vi "Process.vi"(8 "error in":errorcluster, 11 "Instrument.OxfordVRM UI.lvclass":refnum<class "Instrument.OxfordVRM UI.lvclass">) -> (0 "error out":errorcluster, 3 "Instrument.OxfordVRM UI.lvclass":refnum<class "Instrument.OxfordVRM UI.lvclass">)   [LabVIEW 2016, in "Instrument.OxfordVRM UI.lvclass"]
doc: "---------------------------------------------------------------\nJKI State Machine Objects™\nhttp://jki.net/state-machine-objects/\nCopyright (C) 2005-2015, JKI <info@jki.net>\nALL RIGHTS RESERVEDJKI State Machine Objects (SMO) 1.0.0.5\nJKI - JKI\nCopyright (c) 2016, JKI"
uses:
  Instrument.OxfordVRM UI.lvclass
  <vilib>/JKI/JKI SMO/SMO/SMO.lvclass
  <vilib>/JKI/JKI SMO/SMO/Typedefs/Parent Call--Enum.ctl
  <vilib>/JKI/JKI SMO/SMO.UI/SMO.UI.lvclass
  <userlib>/LevyLab/Levylab Instruments/SMOs/Instrument/Instrument.lvclass
  Instrument.OxfordVRM/Typedefs/getAll.ctl
  Instrument.OxfordVRM/Instrument.OxfordVRM.lvclass
  <userlib>/LevyLab/Levylab Instruments/SMOs/Instrument UI/Instrument UI.lvclass
  C:/Program Files (x86)/National Instruments/LabVIEW 2016/user.lib/LevyLab/Levylab Instruments/SMOs/Instrument UI/Instrument UI.lvclass
  C:/Program Files (x86)/National Instruments/LabVIEW 2016/vi.lib/JKI/JKI SMO/SMO.UI/SMO.UI.lvclass
  C:/Program Files (x86)/National Instruments/LabVIEW 2016/vi.lib/JKI/JKI SMO/SMO/SMO.lvclass
  C:/Program Files (x86)/National Instruments/LabVIEW 2016/user.lib/LevyLab/Levylab Instruments/Instrument Types/Cryostat/Instrument.Cryostat.lvclass
  C:/Program Files (x86)/National Instruments/LabVIEW 2016/user.lib/LevyLab/Levylab Instruments/SMOs/Instrument/Instrument.lvclass
panel:
  out "Target Rate (T)":dbl[](array[numeric])
  out "Setpoint (T) (sph)":dbl[](array[numeric])
  in  "Setpoint (T)":dbl[](array[numeric])
  out "Field (T) (sph)":dbl[](array[numeric])
  out "Target Field (T) (sph)":dbl[](array[numeric])
  out "Target Field (T)":dbl[](array[numeric])
  out "Field (T)":dbl[](array[numeric])
  out "XY Graph":cluster{dbl[], dbl[]}[](graph)
  out "XZ Graph":cluster{dbl[], dbl[]}[](graph)
  out "Voltage Meter 6":dbl(knob) scale=-10.0..10.0
  out "Voltage Meter 5":dbl(knob) scale=-10.0..10.0
  out "Voltage Meter 4":dbl(knob) scale=-10.0..10.0
  out "Voltage Meter 3":dbl(knob) scale=-10.0..10.0
  out "Voltage Meter 2":dbl(knob) scale=-10.0..10.0
  out "Current Meter 6":dbl(knob) scale=-120.0..120.0
  out "Current Meter 5":dbl(knob) scale=-120.0..120.0
  out "Current Meter 4":dbl(knob) scale=-120.0..120.0
  out "Current Meter 3":dbl(knob) scale=-120.0..120.0
  out "Current Meter 2":dbl(knob) scale=-120.0..120.0
  out "Voltage Meter 1":dbl(knob) scale=-10.0..10.0
  out "Current Meter 1":dbl(knob) scale=-120.0..120.0
  out "System Time (HH:MM:SS)":dbl=165.3592643737793 format="%<%I:%M:%S %p>T"
  out "ETA":dbl=3660699600.0 format="%<%I:%M:%S %p %m/%d/%Y>T"
  out "version":string="v20/10/28"
  in  "Window Maximize":bool
  in  "Window Minimize":bool
  out "Magnet Status 3":string="Status: Clamped"
  in  "Hold":bool
  in  "To Set":bool
  in  "Export":bool
  in  "Target Field (T)":dbl caption="Field" format="%.2f"
  in  "Target Rate (T/min)":dbl=0.1 caption="Rate" min=0.0 max=1.0 format="%.2f"
  in  "To Zero":bool
  in  "Clamp":bool
  out "Magnet Status 2":string="Status: Clamped"
  in  "Power":bool
  # "Status"
  # "Actions"
  # "Targets"
  # "IPS"
  # "PSU 1 Current (A)"
  # "PSU 1 Voltage (V)"
  # "PSU 2 Current (A)"
  # "PSU 2 Voltage (V)"
  # "PSU 3 Current (A)"
  # "PSU 3 Voltage (V)"
  # "PSU 4 Current (A)"
  # "PSU 4 Voltage (V)"
  # "PSU 5 Current (A)"
  # "PSU 5 Voltage (V)"
  # "PSU 6 Current (A)"
  # "PSU 6 Voltage (V)"
  # "SMO UI Template"
  # "X \t\t\nCurrent (A)\tField (T)\t    Rate (T/min)\n0  - 30 \t   0    - 0.6 \t  0.06\n30 - 42\t    0.6  - 0.85\t  0.048\n42 - 60\t    0.85 - 1.2\t   0.042\n60 - 80\t    1.2  - 1.6\t   0.036\n80 - 99\t    1.6  - 2.0\t   0.024"
  # "Y \t\t\nCurrent (A)\tField (T)\t    Rate (T/min)\n0  - 30\t    0    - 0.6\t   0.048\n30 - 35\t    0.6  - 0.69\t  0.035\n35 - 45\t    0.69 - 0.89\t  0.03\n45 - 60\t    0.89 - 1.2\t   0.024\n60 - 80\t    1.2  - 1.58\t  0.018\n80 - 101\t   1.58 - 2\t     0.01"
  # "Z \t\t\nCurrent (A)\tField (T)\t    Rate (T/min)\n0  - 30\t    0    - 2.6    0.26\n30 - 60\t    2.6  - 5.3\t   0.21\n60 - 80\t    5.3  - 7.1\t   0.16\n80 - 90\t    7.1  - 8\t     0.13\n90 - 101\t   8    - 9\t     0.1\n\n2 OR MORE AXES\n0.005 T/min"
  # "For instructions on how to use the JKI State Machine Objects, examples and video tutorials, visit:\nhttp://jki.net/state-machine-objects/\n\nJKI State Machine Objects™\nhttp://jki.net/state-machine-objects/\nCopyright (C) 2005-2015, JKI <info@jki.net>\nALL RIGHTS RESERVED"
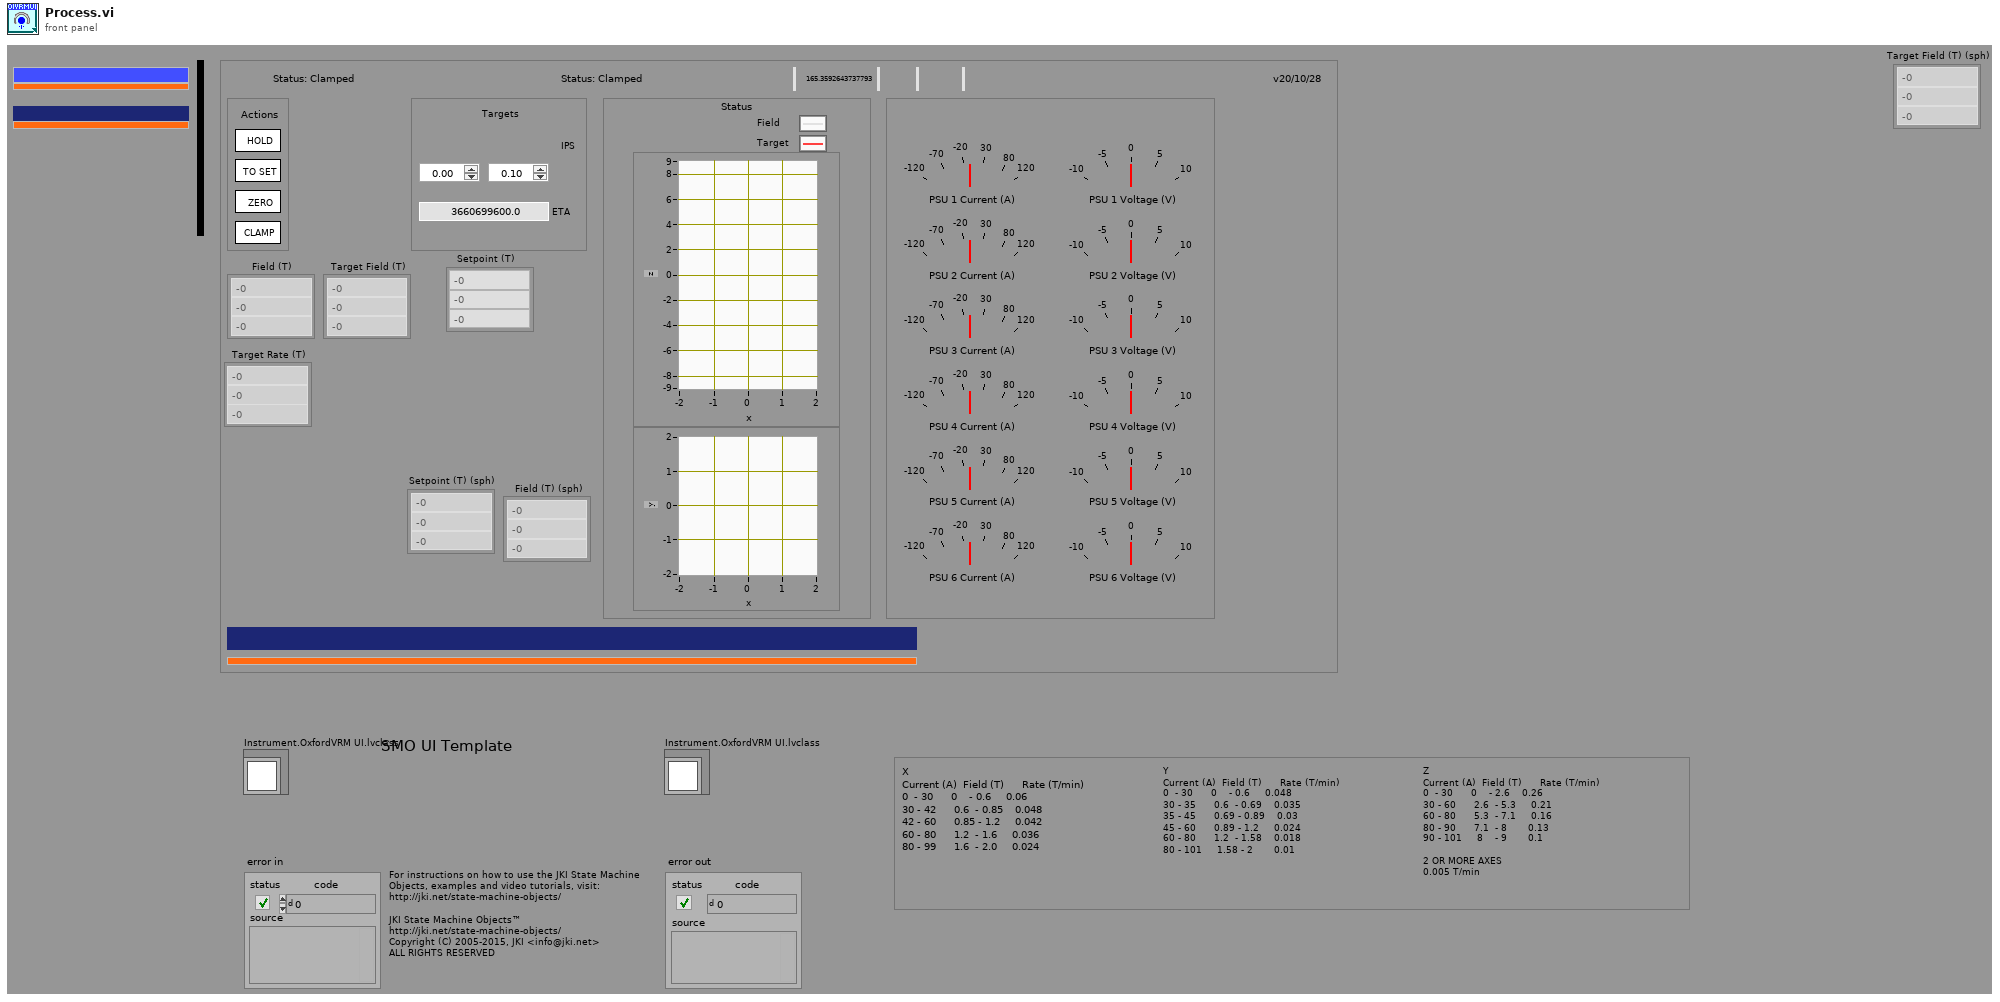
[diagram p1: front panel]
types:
  T1 = typedef "SMO.lvclass/Parent Call--Enum.ctl" = enum16{"Allows parent to run", "Does not request parent to run"}
  T2 = enum32{"invalid app kind", "Development System", "Run Time System", "Student Edition", "Embedded LabVIEW", "Evaluation", "Custom"}
  T3 = typedef "Instrument.OxfordVRM.lvclass/getAll.ctl" = cluster{"Field":dbl[], "Target Field":dbl[], "Target Field Rate":dbl[], "PSU Current":dbl[], "PSU Voltage":dbl[], "Status":string[]}
  T4 = enum32{"Invalid", "Standard", "Closed", "Hidden", "Minimized", "Maximized"}
  T5 = typedef "RemoteControl.lvclass/Message--Cluster.ctl" = cluster{"Command":string, "Data":variant, "Message ID":i32}
  T6 = cluster{"Core":cluster{"Current VI Reference":refnum<vi>, "Close Panel on Exit?":bool, "error":errorcluster}, "Instrument UI out":refnum<class "Instrument.OxfordVRM UI.lvclass">, "Instrument":refnum<class "Instrument.OxfordVRM.lvclass">, "getAll":variant, "Response":string, "config":variant, "switch time":timestamp, "LPF time":timestamp}
  T7 = typedef "Instrument.OxfordVRM.lvclass/PublicEvents--Instrument.Oxford1820.ProcessStatus.ctl" = string
  T8 = cluster{"Current VI Reference":refnum<vi>, "Close Panel on Exit?":bool, "error":errorcluster}
  T9 = typedef "LVRectTypeDef.ctl" = cluster{"Left":i16, "Top":i16, "Right":i16, "Bottom":i16}
  T10 = typedef "SMO.lvclass/Protected Events.ctl" = cluster{"StopProcesses":refnum<user-event>, "AbortProcesses":refnum<user-event>, "Config Changed":refnum<user-event>, "Dependency":refnum<user-event>}
  T11 = typedef "Instrument.lvclass/PublicEvents--Cluster.ctl" = cluster{"MessageFromProcess":refnum<user-event>}
  T12 = typedef "Instrument.OxfordVRM.lvclass/PublicEvents--Cluster.ctl" = cluster{"ProcessStatus":refnum<user-event>}
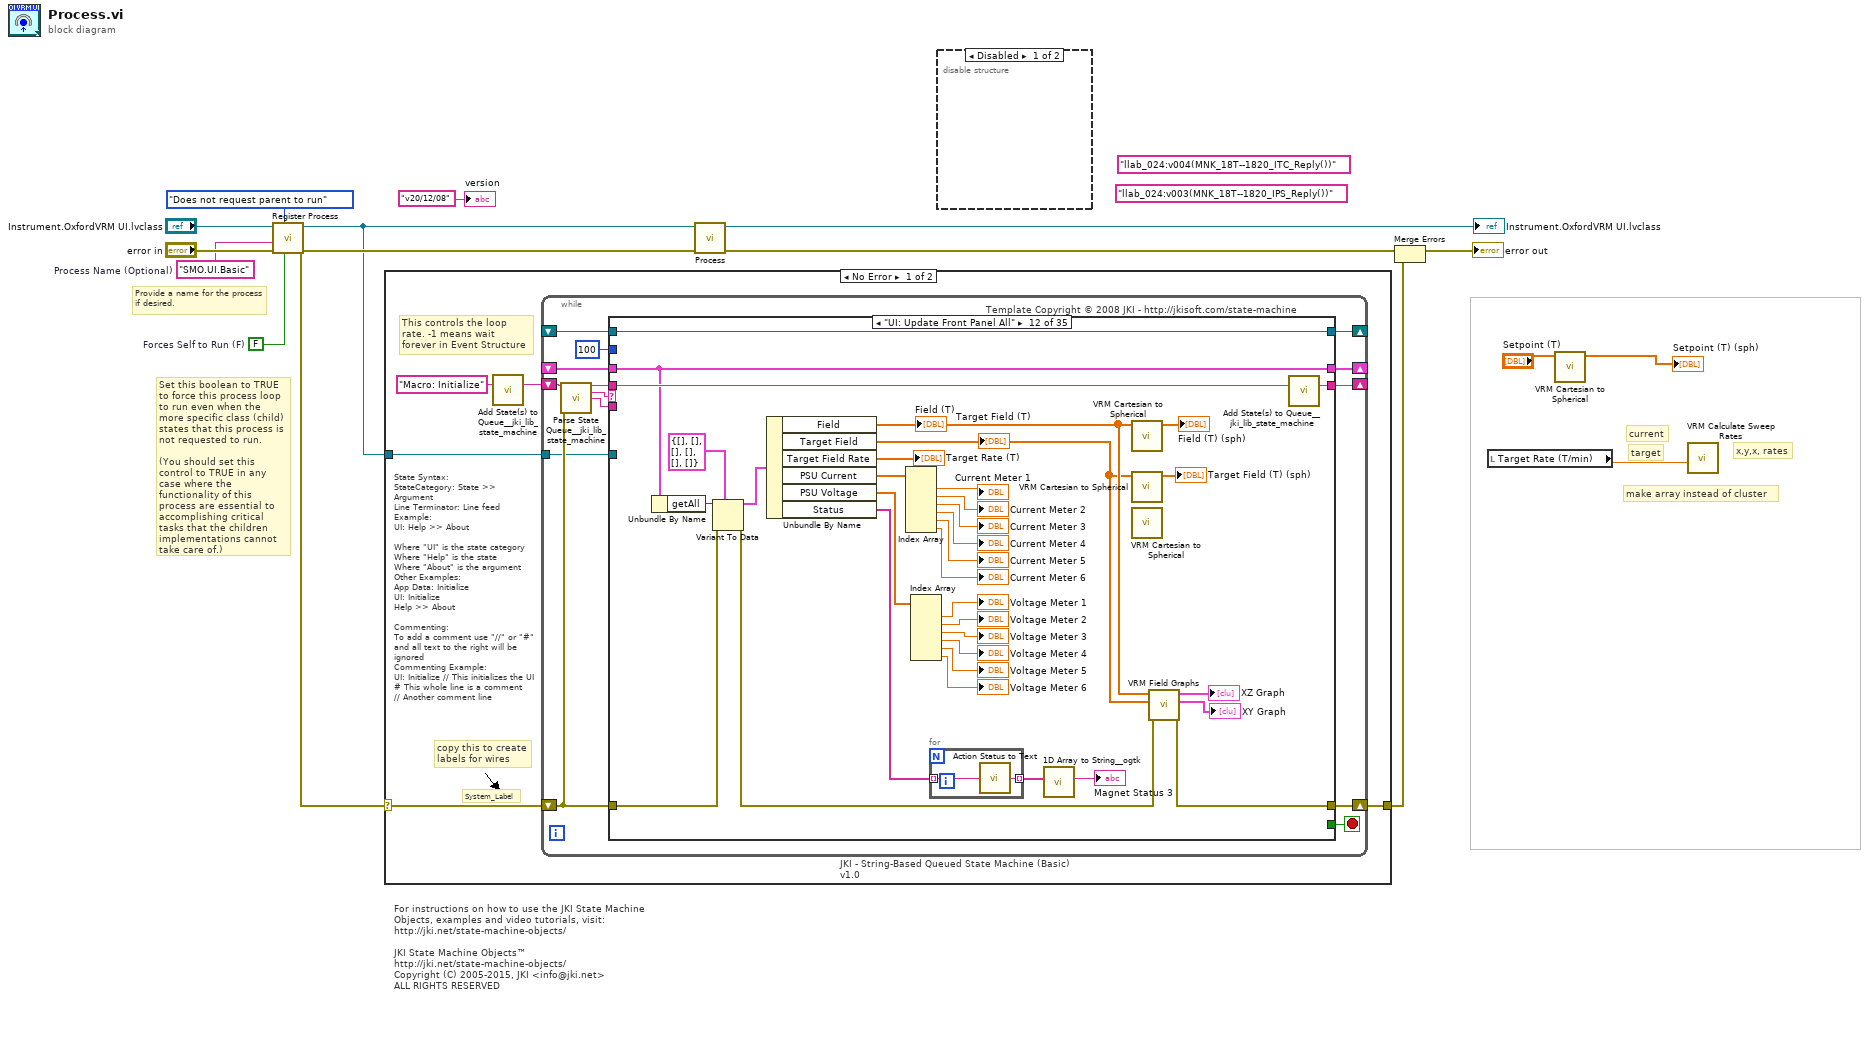
[diagram p0: block diagram]
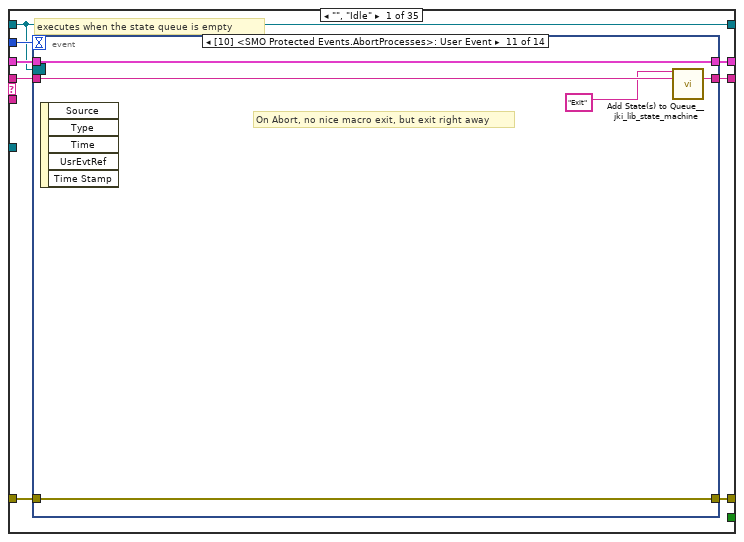
[diagram p3: hidden frame]
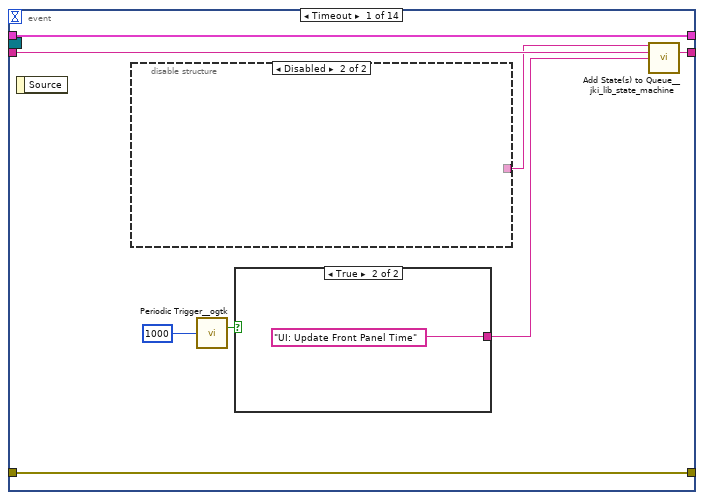
[diagram p4: hidden frame]
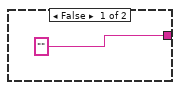
[diagram p5: hidden frame]
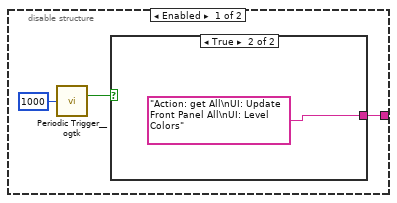
[diagram p6: hidden frame]
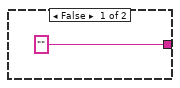
[diagram p7: hidden frame]
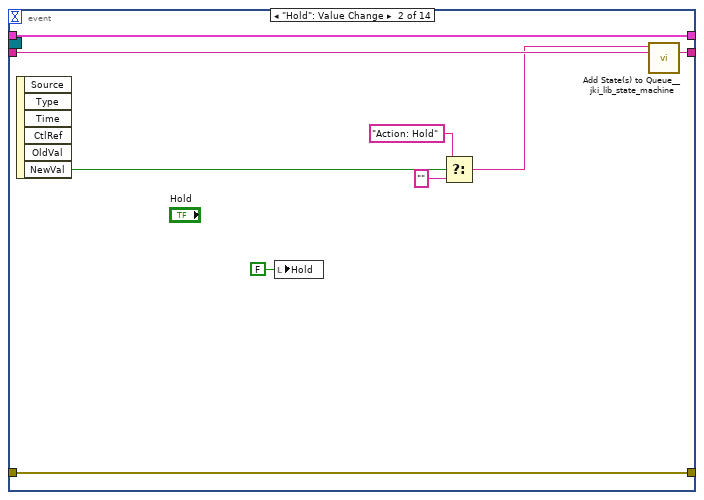
[diagram p8: hidden frame]
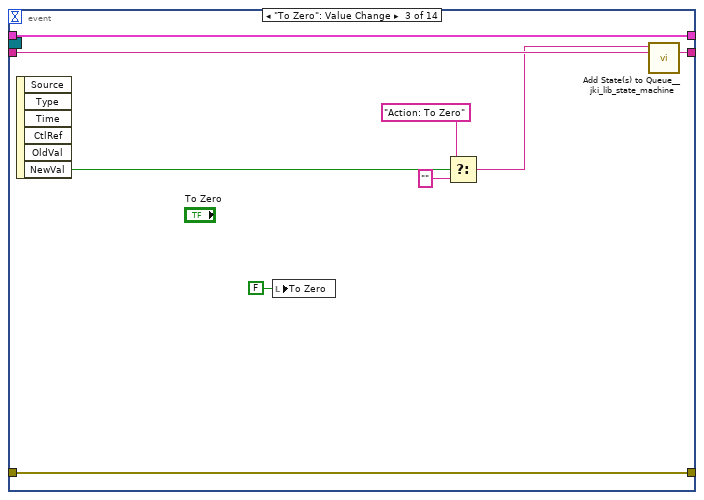
[diagram p9: hidden frame]
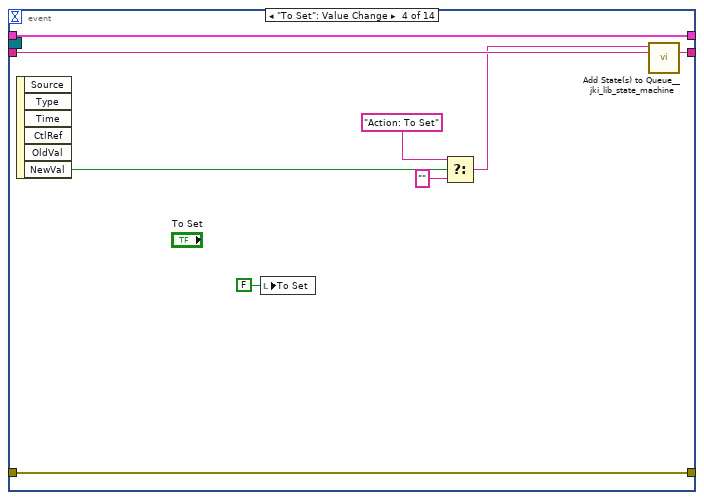
[diagram p10: hidden frame]
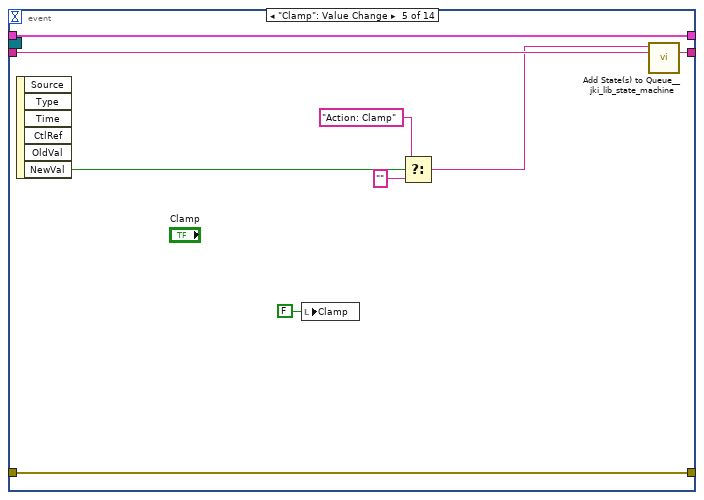
[diagram p11: hidden frame]
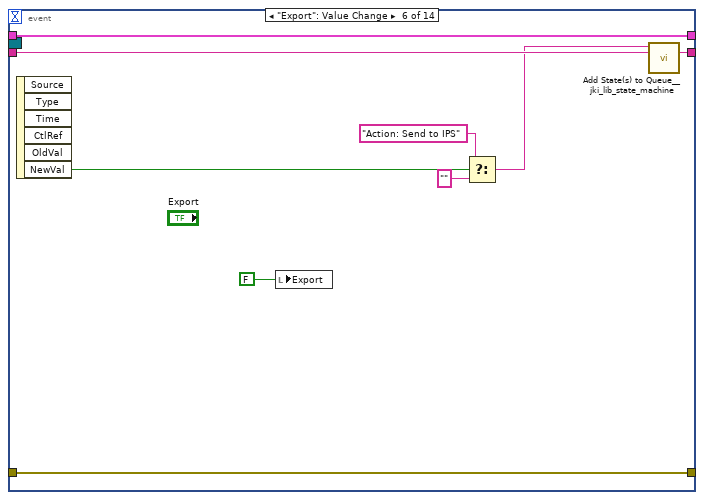
[diagram p12: hidden frame]
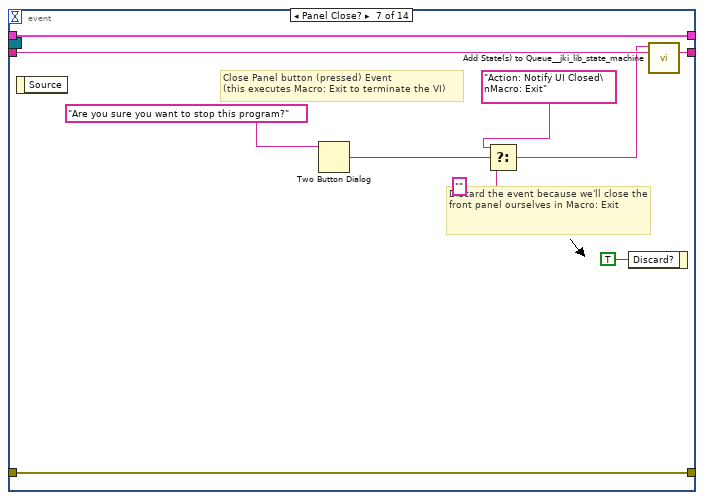
[diagram p13: hidden frame]
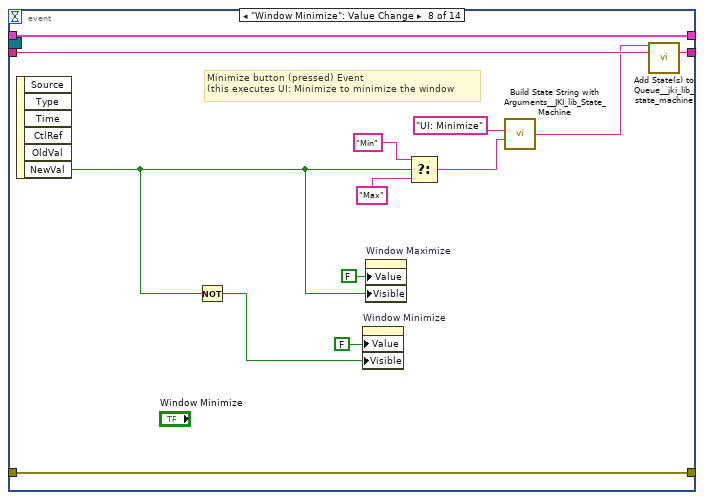
[diagram p14: hidden frame]
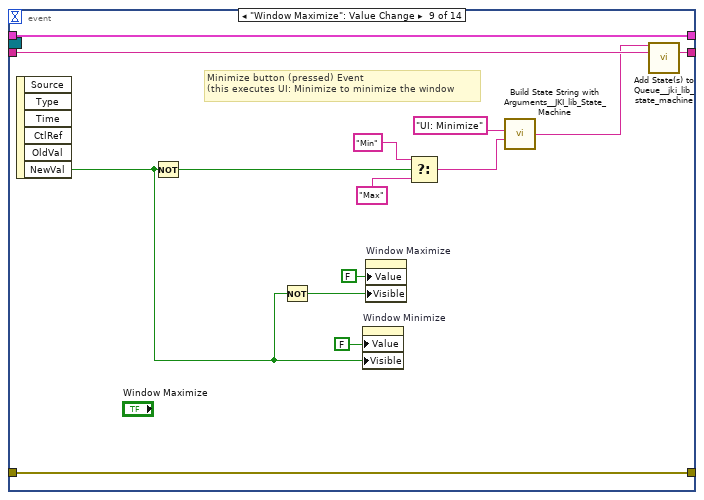
[diagram p15: hidden frame]
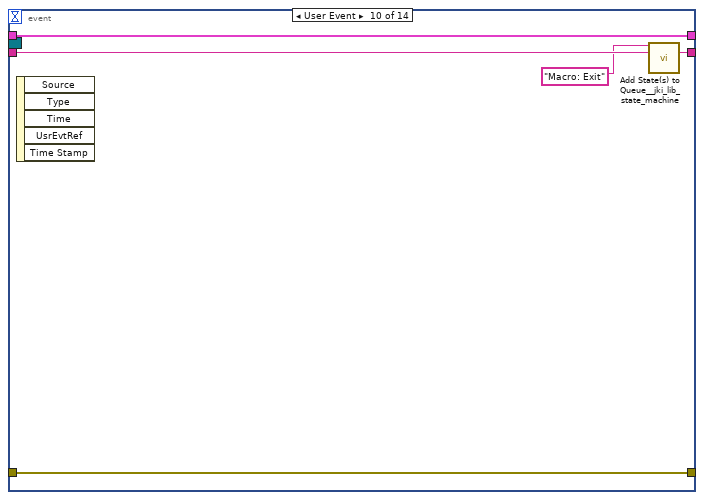
[diagram p16: hidden frame]
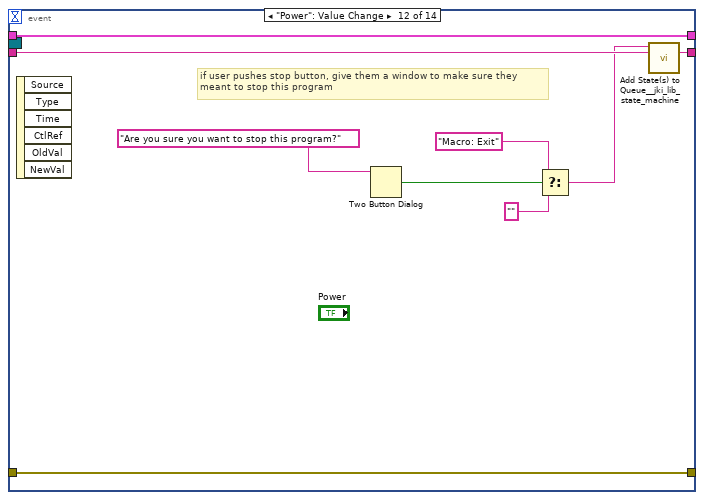
[diagram p17: hidden frame]
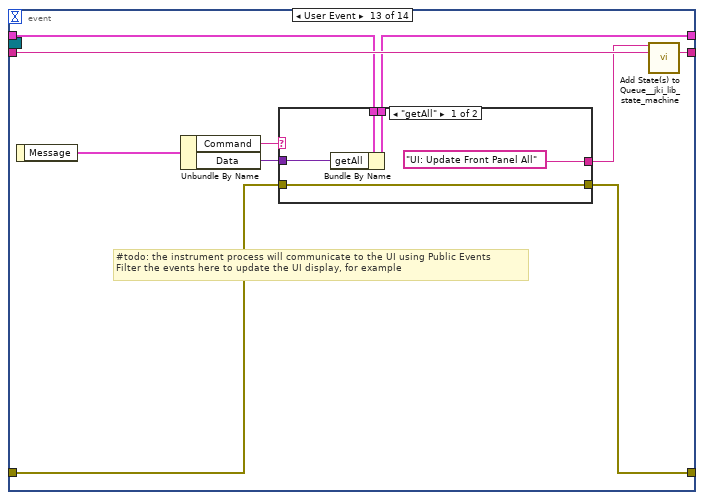
[diagram p18: hidden frame]
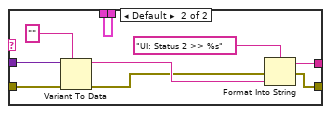
[diagram p19: hidden frame]
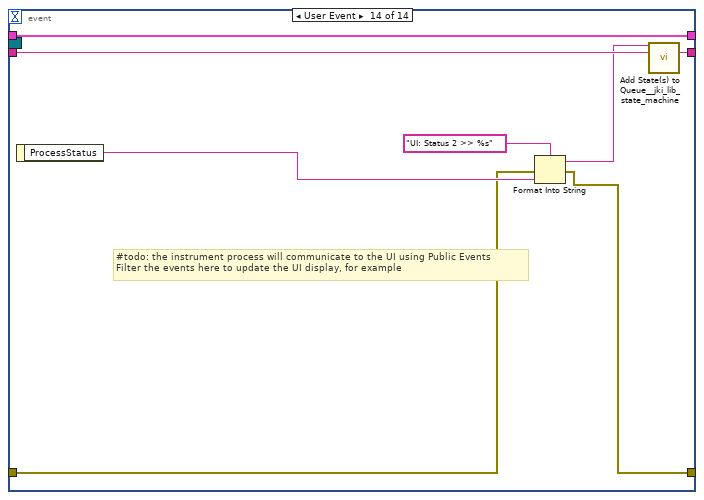
[diagram p20: hidden frame]
diagram:
  (unwired) "llab_024:v004(MNK_18T--1820_ITC_Reply())" ("variable")
  (unwired) "llab_024:v003(MNK_18T--1820_IPS_Reply())" ("variable")
  w6 = FALSE  # Forces Self to Run (F)
  w5 = "SMO.UI.Basic"  # Process Name (Optional)
  # "make array instead of cluster"
  # "x,y,x, rates"
  # "target"
  # "current"
  # "Provide a name for the process\nif desired."
  # "Set this boolean to TRUE to force this process loop to run even when the more specific class (child) states that this process is not requested to run.\n\n(You should set this control to TRUE in any case where the functionality of this process are essential to accomplishing critical tasks that the children implementations cannot take care of.)"
  # "For instructions on how to use the JKI State Machine Objects, examples and video tutorials, visit:\nhttp://jki.net/state-machine-objects/\n\nJKI State Machine Objects™\nhttp://jki.net/state-machine-objects/\nCopyright (C) 2005-2015, JKI <info@jki.net>\nALL RIGHTS RESERVED"
  n1 = call <vilib>:"Register Process.vi"("Forces Self to Run (F)"=w6, "Parent Call"=Parent_Call--Enum."Does not request parent to run", "error in (no error)"="error in", "Process Name (optional)"=w5, "SMO"="Instrument.OxfordVRM UI.lvclass") -> ("error out"=w12:errorcluster, "SMO out"=w11:refnum<class "Instrument.OxfordVRM UI.lvclass">)  [unwired: 5 in]
  n2 = case shown="No Error" w12 {
    selector: w12 -> [w17 w568]
    tunnel: w11 -> [w18 _]
    tunnel: [w16 w568] -> w8
    frame No Error {
      # "State Syntax:\nStateCategory: State >> Argument\nLine Terminator: Line feed\nExample:\nUI: Help >> About\n\nWhere \"UI\" is the state category\nWhere \"Help\" is the state\nWhere \"About\" is the argument\nOther Examples:\nApp Data: Initialize\nUI: Initialize\nHelp >> About\n\nCommenting:\nTo add a comment use \"//\" or \"#\" and all text to the right will be ignored\nCommenting Example:\nUI: Initialize // This initializes the UI\n# This whole line is a comment\n// Another comment line"
      # "copy this to create labels for wires"
      # "This controls the loop rate. -1 means wait forever in Event Structure"
      # "System_Label"
      n3 = call <vilib>:"Add State(s) to Queue__jki_lib_state_machine.vi"("State(s) in (\"\")"="Macro: Initialize") -> ("States Out"=w20:string)  [unwired: 14 in]
      n4 = while "JKI - String-Based Queued State Machine (Basic) v1.0" {
        shift-right: [w27] -> _
        shift-left: _ -> [w26]
        shift-right: [w30] -> w16
        shift-left: w17 -> [w24]
        shift-right: [w29] -> _
        shift-left: w20 -> [w31]
        tunnel: w18 -> [w23]
        shift-right: [w22] -> _
        shift-left: _ -> [w21]
        stop <- w28 stop-if-true
        # "Template Copyright © 2008 JKI - http://jkisoft.com/state-machine"
        n5 = call <vilib>:"Parse State Queue__jki_lib_state_machine.vi"("State Queue"=w31, "Error In (no error)"=w24) -> ("Remaining States"=w33:string, "Current State"=w34:string, "Arguments"=w32:string)  [unwired: 11 in]
        n6 = case shown="\"UI: Update Front Panel All\"" w34 {
          selector: w34 -> [_ _ w197 _ _ _ _ _ _ _ _ _ _ _ _ _ _ _ _ _ _ _ _ _ _ _ _ _ _ _ _ _ _ _ _]
          tunnel: w33 -> [w42 w195 w201 w220 w234 w240 w245 w268 w275 w280 w291 w325 w337 w343 w348 w355 w371 w405 w431 w440 w454 w459 w470 w477 w482 w498 w504 w511 w518 w528 w537 w544 w551 w558 w567]
          tunnel: w32 -> [_ _ _ _ _ _ _ _ _ _ _ _ _ w338 _ w349 w365 w406 _ _ _ _ _ _ _ _ _ _ _ _ _ _ _ _ _]
          tunnel: w26 -> [w40 w192 w199 w211 w222 w236 w242 _ w270 w277 w289 w322 w333 w340 w345 w353 w367 w404 w428 w436 w445 w456 w467 w472 w479 w496 w502 w507 w514 w519 w534 w541 w548 w552 w564]
          tunnel: [w39 w193 w203 w217 w227 w235 w243 w256 w271 w278 w286 w316 w335 w341 w346 w350 w368 w399 w429 w438 w452 w457 w461 w473 w480 w492 w499 w508 w512 w522 w533 w538 w545 w553 w559] -> w30
          tunnel: w24 -> [w38 w193 w202 w217 w223 _ w243 w265 w272 w278 w287 w321 w335 w341 w346 w351 w369 w400 w429 w438 w452 w457 w462 w474 w480 w487 w500 w508 w513 w523 w530 w539 w546 w554 w560]
          tunnel: [w41 w194 w200 w219 w233 w239 w244 w267 w274 w279 w290 w324 w336 w342 w347 w354 w370 w410 w430 w439 w453 w458 w469 w476 w481 w497 w503 w510 w517 w527 w536 w543 w550 w557 w566] -> w29
          tunnel: [_ _ _ _ _ TRUE _ _ _ _ _ _ _ _ _ _ _ _ _ _ _ _ _ _ _ _ _ _ _ _ _ _ _ _ _] -> w28
          tunnel: [w37 w192 w199 w218 w225 w236 w242 w266 w270 w277 w289 w322 w333 w340 w345 w353 w367 w404 w428 w436 w445 w456 w467 w472 w479 w496 w502 w506 w514 w525 w534 w541 w548 w552 w564] -> w27
          tunnel: 100 ("Timeout") -> [w36 _ _ _ _ _ _ _ _ _ _ _ _ _ _ _ _ _ _ _ _ _ _ _ _ _ _ _ _ _ _ _ _ _ _]
          tunnel: w23 -> [_ _ _ _ _ _ _ w253 _ _ _ _ _ _ _ _ _ _ _ _ _ _ _ _ _ _ _ _ _ _ _ _ _ _ _]
          tunnel: [w35 w191 w196 w208 w232 w237 w241 w263 w269 w276 w288 w323 w334 w339 w344 w352 w364 w409 w427 w437 w446 w455 w468 w475 w478 w495 w501 w509 w516 w526 w535 w542 w549 w556 w565] -> w22
          tunnel: w21 -> [w35 w191 w196 w208 w232 w237 w241 w263 w269 w276 w288 w323 w334 w339 w344 w352 w364 w409 w427 w437 w446 w455 w468 w475 w478 _ w501 w509 w516 w526 w535 w542 w549 w556 w565]
          frame "", "Idle" {
            # "executes when the state queue is empty"
            n7 = event shown="[10] <SMO Protected Events.AbortProcesses>: User Event" {
              selector: w35 -> [_ _ _ _ _ _ _ _ _ _ _ _ _ _]
              dyn-events: _ -> [_ _ _ _ _ _ _ _ _ _ _ _ _ _]
              timeout: w36 -> [_ _ _ _ _ _ _ _ _ _ _ _ _ _]
              tunnel: w42 -> [w50 w66 w75 w84 w93 w102 w112 w125 w139 w144 w149 w158 w168 w190]
              tunnel: [w49 w65 w74 w83 w92 w101 w111 w124 w138 w143 w148 w157 w167 w189] -> w41
              tunnel: w40 -> [w46 w63 w72 w81 w90 w99 w109 w123 w137 w141 w146 w155 w166 w183]
              tunnel: [w48 w64 w73 w82 w91 w100 w108 w122 w136 w142 w147 w156 w159 w187] -> w39
              tunnel: w38 -> [w48 w64 w73 w82 w91 w100 w108 w122 w136 w142 w147 w156 w160 w184]
              tunnel: [w46 w63 w72 w81 w90 w99 w109 w123 w137 w141 w146 w155 w165 w183] -> w37
              event Timeout {
                n8 = event-data() -> ()  [unwired: 1 in, 1 out]
                n9 = disable-structure shown="Disabled" {
                  disable-tunnel: [w53 _] -> w47
                  frame Enabled {
                    n10 = call <userlib>:"Periodic Trigger__ogtk.vi"("time (ms)"=u32 1000 ("update time (ms)")) -> ("Triggered"=w55:bool)  [unwired: 12 in, 2 out]
                    n11 = case shown="True" w55 {
                      tunnel: ["" "Action: get All\nUI: Update Front Panel All\nUI: Level Colors"] -> w53
                      frame False {
                      }
                      frame True {
                      }
                    }
                  }
                  frame Disabled {
                  }
                }
                n12 = call <userlib>:"Periodic Trigger__ogtk.vi"("time (ms)"=u32 1000 ("update time (ms)")) -> ("Triggered"=w44:bool)  [unwired: 12 in, 2 out]
                n13 = case shown="True" w44 {
                  tunnel: ["" "UI: Update Front Panel Time"] -> w43
                  frame False {
                  }
                  frame True {
                  }
                }
                n14 = call <vilib>:"Add State(s) to Queue__jki_lib_state_machine.vi"("State(s) in Front (\"\")"=w47, "State(s) in (\"\")"=w50, "State(s) at Back (\"\")"=w43) -> ("States Out"=w49:string)  [unwired: 12 in]
              }
              event "Hold": Value Change {
                n15 = event-data() -> ("NewVal"=w62:bool)  [unwired: 1 in, 5 out]
                n16 = local write "Hold"(FALSE ("Hold")) -> ()
                n17 = Select(t="Action: Hold" ("State(s) in Front (\"\")"), s=w62, f="") -> (s? t:f=w59:string)
                n18 = call <vilib>:"Add State(s) to Queue__jki_lib_state_machine.vi"("State(s) in Front (\"\")"=w59, "State(s) in (\"\")"=w66) -> ("States Out"=w65:string)  [unwired: 13 in]
              }
              event "To Zero": Value Change {
                n19 = event-data() -> ("NewVal"=w70:bool)  [unwired: 1 in, 5 out]
                n20 = local write "To Zero"(FALSE ("To Zero")) -> ()
                n21 = Select(t="Action: To Zero" ("State(s) in Front (\"\")"), s=w70, f="") -> (s? t:f=w68:string)
                n22 = call <vilib>:"Add State(s) to Queue__jki_lib_state_machine.vi"("State(s) in Front (\"\")"=w68, "State(s) in (\"\")"=w75) -> ("States Out"=w74:string)  [unwired: 13 in]
              }
              event "To Set": Value Change {
                n23 = event-data() -> ("NewVal"=w79:bool)  [unwired: 1 in, 5 out]
                n24 = local write "To Set"(FALSE ("To Set")) -> ()
                n25 = Select(t="Action: To Set" ("State(s) in Front (\"\")"), s=w79, f="") -> (s? t:f=w77:string)
                n26 = call <vilib>:"Add State(s) to Queue__jki_lib_state_machine.vi"("State(s) in Front (\"\")"=w77, "State(s) in (\"\")"=w84) -> ("States Out"=w83:string)  [unwired: 13 in]
              }
              event "Clamp": Value Change {
                n27 = event-data() -> ("NewVal"=w88:bool)  [unwired: 1 in, 5 out]
                n28 = local write "Clamp"(FALSE ("Clamp")) -> ()
                n29 = Select(t="Action: Clamp" ("State(s) in Front (\"\")"), s=w88, f="") -> (s? t:f=w86:string)
                n30 = call <vilib>:"Add State(s) to Queue__jki_lib_state_machine.vi"("State(s) in Front (\"\")"=w86, "State(s) in (\"\")"=w93) -> ("States Out"=w92:string)  [unwired: 13 in]
              }
              event "Export": Value Change {
                n31 = event-data() -> ("NewVal"=w98:bool)  [unwired: 1 in, 5 out]
                n32 = local write "Export"(FALSE ("Send to IPS")) -> ()
                n33 = Select(t="Action: Send to IPS" ("State(s) in Front (\"\")"), s=w98, f="") -> (s? t:f=w95:string)
                n34 = call <vilib>:"Add State(s) to Queue__jki_lib_state_machine.vi"("State(s) in Front (\"\")"=w95, "State(s) in (\"\")"=w102) -> ("States Out"=w101:string)  [unwired: 13 in]
              }
              event Panel Close? {
                # "Discard the event because we'll close the front panel ourselves in Macro: Exit"
                # "Close Panel button (pressed) Event\n(this executes Macro: Exit to terminate the VI)"
                n35 = event-data() -> ()  [unwired: 1 in, 1 out]
                n36 = Two Button Dialog(message="Are you sure you want to stop this program?") -> (T button?=w107:bool)  [unwired: 2 in]
                n37 = Select(t="Action: Notify UI Closed\nMacro: Exit", s=w107, f="") -> (s? t:f=w103:string)
                n38 = event-data("Discard?"=TRUE) -> ()  [unwired: 1 in, 1 out]
                n39 = call <vilib>:"Add State(s) to Queue__jki_lib_state_machine.vi"("State(s) in Front (\"\")"=w103, "State(s) in (\"\")"=w112) -> ("States Out"=w111:string)  [unwired: 13 in]
              }
              event "Window Minimize": Value Change {
                # "Minimize button (pressed) Event\n(this executes UI: Minimize to minimize the window"
                n40 = event-data() -> ("NewVal"=w113:bool)  [unwired: 1 in, 5 out]
                n41 = Not(x=w113) -> (.not. x?=w114:bool)
                n42 = property on="Window Minimize" class="Bool (strict)"("Value"=FALSE ("Window Maximize"), "Visible"=w114) -> ()  [unwired: 2 in, 2 out]
                n43 = property on="Window Maximize" class="Bool (strict)"("Value"=FALSE ("Window Maximize"), "Visible"=w113) -> ()  [unwired: 2 in, 2 out]
                n44 = Select(t="Min" ("Arguments (\"\")"), s=w113, f="Max" ("Arguments (\"\")")) -> (s? t:f=w118:string)
                n45 = call <vilib>:"Build State String with Arguments__JKI_lib_State_Machine.vi"("Arguments (\"\")"=w118, "State"="UI: Minimize") -> ("State with Arguments"=w117:string)  [unwired: 4 in]
                n46 = call <vilib>:"Add State(s) to Queue__jki_lib_state_machine.vi"("State(s) in Front (\"\")"=w117, "State(s) in (\"\")"=w125) -> ("States Out"=w124:string)  [unwired: 13 in]
              }
              event "Window Maximize": Value Change {
                # "Minimize button (pressed) Event\n(this executes UI: Minimize to minimize the window"
                n47 = event-data() -> ("NewVal"=w127:bool)  [unwired: 1 in, 5 out]
                n48 = Not(x=w127) -> (.not. x?=w128:bool)
                n49 = Not(x=w127) -> (.not. x?=w126:bool)
                n50 = property on="Window Minimize" class="Bool (strict)"("Value"=FALSE ("Window Maximize"), "Visible"=w127) -> ()  [unwired: 2 in, 2 out]
                n51 = property on="Window Maximize" class="Bool (strict)"("Value"=FALSE ("Window Maximize"), "Visible"=w126) -> ()  [unwired: 2 in, 2 out]
                n52 = Select(t="Min" ("Arguments (\"\")"), s=w128, f="Max" ("Arguments (\"\")")) -> (s? t:f=w132:string)
                n53 = call <vilib>:"Build State String with Arguments__JKI_lib_State_Machine.vi"("Arguments (\"\")"=w132, "State"="UI: Minimize") -> ("State with Arguments"=w131:string)  [unwired: 4 in]
                n54 = call <vilib>:"Add State(s) to Queue__jki_lib_state_machine.vi"("State(s) in Front (\"\")"=w131, "State(s) in (\"\")"=w139) -> ("States Out"=w138:string)  [unwired: 13 in]
              }
              event User Event {
                n55 = event-data() -> ()  [unwired: 1 in, 5 out]
                n56 = call <vilib>:"Add State(s) to Queue__jki_lib_state_machine.vi"("State(s) in Front (\"\")"="Macro: Exit", "State(s) in (\"\")"=w144) -> ("States Out"=w143:string)  [unwired: 13 in]
              }
              event User Event {
                # "On Abort, no nice macro exit, but exit right away"
                n57 = event-data() -> ()  [unwired: 1 in, 5 out]
                n58 = call <vilib>:"Add State(s) to Queue__jki_lib_state_machine.vi"("State(s) in Front (\"\")"="Exit", "State(s) in (\"\")"=w149) -> ("States Out"=w148:string)  [unwired: 13 in]
              }
              event "Power": Value Change {
                # "if user pushes stop button, give them a window to make sure they\nmeant to stop this program"
                n59 = event-data() -> ()  [unwired: 1 in, 6 out]
                n60 = Two Button Dialog(message="Are you sure you want to stop this program?") -> (T button?=w154:bool)  [unwired: 2 in]
                n61 = Select(t="Macro: Exit", s=w154, f="") -> (s? t:f=w150:string)
                n62 = call <vilib>:"Add State(s) to Queue__jki_lib_state_machine.vi"("State(s) in Front (\"\")"=w150, "State(s) in (\"\")"=w158) -> ("States Out"=w157:string)  [unwired: 13 in]
              }
              event User Event {
                # "#todo: the instrument process will communicate to the UI using Public Events\nFilter the events here to update the UI display, for example"
                n63 = event-data() -> ("Message"=w161:T5)  [unwired: 1 in]
                n64 = Unbundle By Name(w161) -> ("Command"=w163:string, "Data"=w164:variant)
                n65 = case shown="\"getAll\"" w163 {
                  tunnel: w164 -> [w173 w181]
                  tunnel: w166 -> [w172 w182]
                  tunnel: [w171 w182] -> w165
                  tunnel: ["UI: Update Front Panel All" w178] -> w162
                  tunnel: w160 -> [w169 w175]
                  tunnel: [w169 w174] -> w159
                  frame "getAll" {
                    n66 = Bundle By Name(cluster=w172, "getAll"=w173) -> (w171:T6)
                  }
                  frame Default {
                    n67 = Variant To Data(error in=w175, type="", Variant=w181) -> (data=w177:string, error out=w176:errorcluster)
                    n68 = Format Into String(format string="UI: Status 2 >> %s", error in=w176, w177) -> (resulting string=w178:string, error out=w174:errorcluster)  [unwired: 1 in]
                  }
                }
                n69 = call <vilib>:"Add State(s) to Queue__jki_lib_state_machine.vi"("State(s) in Front (\"\")"=w162, "State(s) in (\"\")"=w168) -> ("States Out"=w167:string)  [unwired: 13 in]
              }
              event User Event {
                # "#todo: the instrument process will communicate to the UI using Public Events\nFilter the events here to update the UI display, for example"
                n70 = event-data() -> ("ProcessStatus"=w185:T7)  [unwired: 1 in]
                n71 = Format Into String(format string="UI: Status 2 >> %s", error in=w184, w185) -> (resulting string=w188:string, error out=w187:errorcluster)  [unwired: 1 in]
                n72 = call <vilib>:"Add State(s) to Queue__jki_lib_state_machine.vi"("State(s) in Front (\"\")"=w188, "State(s) in (\"\")"=w190) -> ("States Out"=w189:string)  [unwired: 13 in]
              }
            }
          }
          frame "---------- Core ----------" {
            # "Do not put any code in this frame.\n(it is a separator no-op)"
            n73 = call <vilib>:"Add State(s) to Queue__jki_lib_state_machine.vi"("State(s) in (\"\")"=w195) -> ("States Out"=w194:string)  [unwired: 14 in]
          }
          frame Default {
            w206 = 42 items=["No error", "Argument error", "Memory is full", "Out of zone", "End of file", "File already open", "Generic file I/O error", "File not found", "File permission error", "Disk is full", "Duplicate path", "Too many files open", "System feature not enabled", "Resource file not found", "Cannot add resource", "Resource not found", "Image not found", "Image memory error", "Pen does not exist", "Config type invalid", "Config token not found", "Config parse error", "Config memory error", "Bad external code format", "Bad external code offset", "External code not present", "Null window", "Destroy window error", "Null menu", "Print aborted", "Bad print record", "Print driver error", "Windows error during printing", "Memory error during printing", "Print dialog error", "Generic print error", "Invalid device refnum", "Device not found", "Device parameter error", "Device unit error", "Cannot open device", "Device call aborted", "Generic error", "Cancelled by user", "Object ID too low", "Object ID too high", "Object not in heap", "Unknown heap", "Unknown object (invalid DefProc)", "Unknown object (DefProc not in table)", "Message out of range", "Invalid (null) method", "Unknown message", "Manager call not supported", "Bad address", "Network operation in progress", "Network operation timed out", "Connection is busy", "Network attribute not supported", "Network error", "Address in use", "System out of memory", "Connection aborted", "Connection refused", "Not connected", "Already connected", "Connection closed", "Initialization error (interapplication manager)", "Bad occurrence", "Wait on unbound occurrence handler", "Occurrence queue overflow", "Datalog type conflict", "Unused", "Unrecognized type (interapplication manager)", "Memory corrupt", "Failed to make temporary DLL", "Old CIN version", "Drag socket not found", "Failed to load drop-object", "Failed to register OLE object", "Failed to release OLE object", "Format specifier type mismatch", "Unknown format specifier", "Too few format specifiers", "Too many format specifiers", "Scan failed", "Newer CIN version", "Error converting to variant", "Runtime menu error", "Password tampered", "Variant attribute not found", "Incompatible variant data type", "Event data is not available", "Event Store is not present", "Occurrence is not found", "Event Queue is not created", "Event info is not available", "Refnum passed is NULL", "Error retrieving Class GUID", "Error retrieving CoClass GUID", "Error retrieving TypeLib GUID.", "Bad built application magic bytes.", "Specific driver is different from the specific driver associated with the Logical Name.", "There is no session opened to the class driver.", "Max Error", "MAX - Error with config objects", "MAX - Error loading configuration", "MAX - Group not supported"]
            # "Current State"
            # "Do not delete, rename, or modify this frame.\n(this is used to capture unhandled states and typos)"
            # "Handle mistyped state name (developer tool)"
            n74 = Format Into String(format string="Software Exception: Unhandled State \"%s\"." ("message"), error in=w202, w197) -> (resulting string=w205:string, error out=w204:errorcluster)  [unwired: 1 in]
            n75 = call <vilib>:"Error Cluster From Error Code.vi"("show call chain? (False)"=TRUE, "error in (no error)"=w204, "error message (\"\")"=w205, "error code (0)"=w206) -> ("error out"=w203:errorcluster)  [unwired: 5 in]
            n76 = call <vilib>:"Add State(s) to Queue__jki_lib_state_machine.vi"("State(s) in (\"\")"=w201) -> ("States Out"=w200:string)  [unwired: 14 in]
          }
          frame "Initialize Core Data" {
            # "Do not delete, rename, or modify this frame.\n(this is used to determine panel behavior on exit)"
            # "originally closed?"
            # "exe?"
            # "If panel starts closed or is an EXE, then close it when we exit"
            n77 = property class="VI"() -> ("Front Panel.Open"=w216:bool)  [unwired: 2 in, 2 out]
            n78 = property class="App"() -> ("App.Kind"=w215:T2)  [unwired: 2 in, 2 out]
            n79 = control-ref of="Current VI Reference"() -> (w209:refnum<vi>)
            n80 = Not(x=w216) -> (.not. x?=w213:bool)
            n81 = Equal?(x=w215, y=T2."Run Time System" ("Application:Kind")) -> (x = y?=w212:bool)
            n82 = Or(x=w213, y=w212) -> (x .or. y?=w210:bool)
            n83 = Bundle By Name(cluster=w211, "Core.Current VI Reference"=w209, "Core.Close Panel on Exit?"=w210) -> (w218:T6)
            n84 = call <vilib>:"Add State(s) to Queue__jki_lib_state_machine.vi"("State(s) in (\"\")"=w220) -> ("States Out"=w219:string)  [unwired: 14 in]
          }
          frame "Error Handler" {
            w227 = errorcluster {"status"=FALSE, "code"=0, "source"=""}  # No error
            # "Overwrite this method to handle errors and pass to parent if not handled. Parent will fire a public event if the error is not handled up the chain of classes."
            # "Handle any errors here.\nYou can also output any states to clean-up after errors occur"
            n85 = Unbundle By Name(w222) -> ("Instrument UI out"=w231:refnum<class "Instrument.OxfordVRM UI.lvclass">)
            n86 = call-dynamic "Handle Error.vi"("Stop on Unhandled Error (T)"=FALSE, "error in"=w223, "Instrument.Oxford1820 UI"=w231) -> ("handling error"=w221:errorcluster, "Unhandled error"=w226:errorcluster)  [unwired: 6 in, 1 out]
            n87 = Bundle By Name(cluster=w222, "Core.error"=w226) -> (w225:T6)
            n88 = Select(t="Exit", s=w221, f="") -> (s? t:f=w228:string)
            n89 = call <vilib>:"Add State(s) to Queue__jki_lib_state_machine.vi"("State(s) in Front (\"\")"=w228, "State(s) in (\"\")"=w234) -> ("States Out"=w233:string)  [unwired: 13 in]
          }
          frame "Exit" {
            # "Do not put any code in this frame.\n(No errors that occur here will be handled.)"
            n90 = Unbundle By Name(w236) -> ("Core.error"=w235:errorcluster)
            n91 = call <vilib>:"Add State(s) to Queue__jki_lib_state_machine.vi"("State(s) in (\"\")"=w240) -> ("States Out"=w239:string)  [unwired: 14 in]
          }
          frame "---------- Data ----------" {
            # "Do not put any code in this frame.\n(It is a separator no-op. You can make a copy of this frame to create a new Data frame)"
            n92 = call <vilib>:"Add State(s) to Queue__jki_lib_state_machine.vi"("State(s) in (\"\")"=w245) -> ("States Out"=w244:string)  [unwired: 14 in]
          }
          frame "Data: Initialize" {
            w246 = refnum<class "Instrument.OxfordVRM.lvclass"> refnum  # Instrument
            w254 = timestamp(0 s since 1904-01-01)  # LPF time
            w258 = timestamp(0 s since 1904-01-01)  # switch time
            w259 = variant  # config
            w260 = ""  # Response
            w261 = variant  # getAll
            w262 = T8 {"Current VI Reference"=refnum, "Close Panel on Exit?"=FALSE, "error"={"status"=FALSE, "code"=0, "source"=""}}  # Core
            w264 = refnum<class "Instrument.OxfordVRM UI.lvclass"> refnum  # Self Reference
            # "do not delete - used by framework"
            # "Data names and types of shift register data are defined by this bundle."
            # "Initialize the shift-register data, here.\n(data names are defined by what you wire into the bundle function)"
            n93 = Variant To Data(error in=w265, type=w264, Variant=w253) -> (data=w252:refnum<class "Instrument.OxfordVRM UI.lvclass">, error out=w251:errorcluster)
            n94 = call <userlib>:"Read Instrument.vi"("error in (no error)"=w251, "Instrument UI in"=w252) -> ("error out"=w250:errorcluster, "Instrument.lvclass"=w247:refnum<class "Instrument.lvclass">, "Instrument UI out"=w248:refnum<class "Instrument.OxfordVRM UI.lvclass">)  [unwired: 7 in]
            n95 = To More Specific Class(target class=w246, reference=w247) -> (specific class reference=w249:refnum<class "Instrument.OxfordVRM.lvclass">)  [unwired: 1 in, 1 out]
            n96 = Get Date/Time In Seconds() -> (seconds since 1Jan1904=w257:timestamp)
            n97 = Variant To Data(error in=w250, type=w258, Variant=w257) -> (data=w255:timestamp, error out=w256:errorcluster)
            n98 = Bundle("Core"=w262, "Instrument UI out"=w248, "Instrument"=w249, "getAll"=w261, "Response"=w260, "config"=w259, "switch time"=w255, "LPF time"=w254) -> (w266:T6)  [unwired: 1 in]
            n99 = call <vilib>:"Add State(s) to Queue__jki_lib_state_machine.vi"("State(s) in (\"\")"=w268) -> ("States Out"=w267:string)  [unwired: 14 in]
          }
          frame "Data: Cleanup" {
            # "Cleanup any data and references, here.\n(this is called automatically, by the Macro: Exit)"
            n100 = Unbundle By Name(w270) -> ("Core.Current VI Reference"=w273:refnum<vi>)
            n101 = Close Reference(reference=w273, error in (no error)=w272) -> (error out=w271:errorcluster)
            n102 = call <vilib>:"Add State(s) to Queue__jki_lib_state_machine.vi"("State(s) in (\"\")"=w275) -> ("States Out"=w274:string)  [unwired: 14 in]
          }
          frame "---------- UI ----------" {
            # "Do not put any code in this frame.\n(It is a separator no-op. You can make a copy of this frame to create a new UI frame)"
            n103 = call <vilib>:"Add State(s) to Queue__jki_lib_state_machine.vi"("State(s) in (\"\")"=w280) -> ("States Out"=w279:string)  [unwired: 14 in]
          }
          frame "UI: Initialize" {
            # "size window to decoration box on front panel"
            # "Initialize the User Interface, here.\n(this is called automatically, by the Macro: Init)"
            n104 = property on="Window Minimize" class="Bool (strict)"("Value"=FALSE ("Window Maximize"), "Visible"=TRUE ("Window Maximize")) -> ()  [unwired: 2 in, 2 out]
            n105 = property on="Window Maximize" class="Bool (strict)"("Value"=FALSE ("Window Maximize"), "Visible"=FALSE ("Window Maximize")) -> ()  [unwired: 2 in, 2 out]
            n106 = invoke on="Power" class="Bool (strict)" method="Reinit To Default"() -> ()  [unwired: 3 in, 3 out]
            n107 = call <userlib>:"Fit VI window to Largest Dec__ogtk.vi"("error in (no error)"=w287, "border spacing (2 px)"=0) -> ("error out"=w286:errorcluster)  [unwired: 4 in, 1 out]
            n108 = call <vilib>:"Add State(s) to Queue__jki_lib_state_machine.vi"("State(s) in (\"\")"=w291) -> ("States Out"=w290:string)  [unwired: 14 in]
          }
          frame "UI: Update Front Panel All" {
            n109 = Unbundle By Name(w322) -> ("getAll"=w320:variant)
            n110 = Variant To Data(error in=w321, type=T3 {"Field"=[], "Target Field"=[], "Target Field Rate"=[], "PSU Current"=[], "PSU Voltage"=[], "Status"=[]} ("getAll"), Variant=w320) -> (data=w318:T3, error out=w317:errorcluster)
            n111 = Unbundle By Name(w318) -> ("Field"=w310:dbl[], "Target Field"=w309:dbl[], "Target Field Rate"=→"Target Rate (T)":dbl[], "PSU Current"=w292:dbl[], "PSU Voltage"=w293:dbl[], "Status"=w295:string[])
            "Field (T)" <- w310
            "Target Field (T)" <- w309
            n112 = Index Array(array=w292) -> (element #1=→"Current Meter 1":dbl, element #2=→"Current Meter 2":dbl, element #3=→"Current Meter 3":dbl, element #4=→"Current Meter 4":dbl, element #5=→"Current Meter 5":dbl, element #6=→"Current Meter 6":dbl)  [unwired: 6 in]
            n113 = Index Array(array=w293) -> (element #1=→"Voltage Meter 1":dbl, element #2=→"Voltage Meter 2":dbl, element #3=→"Voltage Meter 3":dbl, element #4=→"Voltage Meter 4":dbl, element #5=→"Voltage Meter 5":dbl, element #6=→"Voltage Meter 6":dbl)  [unwired: 6 in]
            n114 = for {
              tunnel: [w327] -> w311 mode=indexing
              tunnel: w295 -> [w326] mode=indexing
              n115 = call "Action Status to Text.vi"("PSU Act Stat"=w326) -> ("Status:"=w327:string)
            }
            n116 = call <userlib>:"1D Array to String__ogtk.vi"("Array of Strings"=w311) -> ("delimited string"=→"Magnet Status 3":string)  [unwired: 10 in]
            n117 = call "VRM Cartesian to Spherical.vi"("Field (x,y,z)"=w310) -> ("Field (r,theta,phi)"=→"Field (T) (sph)":dbl[])  [unwired: 9 in, 1 out]
            n118 = call "VRM Cartesian to Spherical.vi"("Field (x,y,z)"=w309) -> ("Field (r,theta,phi)"=→"Target Field (T) (sph)":dbl[])  [unwired: 9 in, 1 out]
            n119 = call "VRM Cartesian to Spherical.vi"() -> ()  [unwired: 10 in, 2 out]
            n120 = call "VRM Field Graphs.vi"("error in (no error)"=w317, "Target Field (T)"=w309, "Field (T)"=w310) -> ("error out"=w316:errorcluster, "XY Graph"=→"XY Graph":cluster{dbl[], dbl[]}[], "XZ Graph"=→"XZ Graph":cluster{dbl[], dbl[]}[])  [unwired: 6 in]
            n121 = call <vilib>:"Add State(s) to Queue__jki_lib_state_machine.vi"("State(s) in (\"\")"=w325) -> ("States Out"=w324:string)  [unwired: 14 in]
          }
          frame "UI: Update Front Panel Time" {
            # "Do not put any code in this frame.\n(It is a separator no-op. You can make a copy of this frame to create a new UI frame)"
            n122 = local read "Target Field (T)"() -> (w332:dbl)
            n123 = Get Date/Time In Seconds() -> (seconds since 1Jan1904=w331:timestamp)
            n124 = To Double Precision Float(number=w331) -> (double precision float=→"System Time (HH:MM:SS)":dbl)
            n125 = call "Calculate Sweep ETA.vi"("Target Field (T)"=w332) -> ("ETA timestamp"=w329:timestamp)  [unwired: 8 in, 2 out]
            n126 = To Double Precision Float(number=w329) -> (double precision float=→"ETA":dbl)
            n127 = call <vilib>:"Add State(s) to Queue__jki_lib_state_machine.vi"("State(s) in (\"\")"=w337) -> ("States Out"=w336:string)  [unwired: 14 in]
          }
          frame "UI: Status 2" {
            # "Do not put any code in this frame.\n(It is a separator no-op. You can make a copy of this frame to create a new UI frame)"
            n128 = call <vilib>:"Add State(s) to Queue__jki_lib_state_machine.vi"("State(s) in (\"\")"=w343) -> ("States Out"=w342:string)  [unwired: 14 in]
            "Magnet Status 2" <- w338
          }
          frame "UI: Level Colors" {
            # "Do not put any code in this frame.\n(It is a separator no-op. You can make a copy of this frame to create a new UI frame)"
            n129 = call <vilib>:"Add State(s) to Queue__jki_lib_state_machine.vi"("State(s) in (\"\")"=w348) -> ("States Out"=w347:string)  [unwired: 14 in]
          }
          frame "UI: Cursor Set" {
            # "Argument"
            # "Initialize the User Interface, here.\n(this is called automatically, by the Macro: Init)"
            n130 = disable-structure shown="Default" {
              disable-tunnel: w351 -> [w356 w359]
              disable-tunnel: [w356 w358] -> w350
              disable-tunnel: w349 -> [_ w357]
              frame condition #0 {
              }
              frame condition #1 (active) {
                n131 = case shown="\"Idle\", Default" w357 {
                  tunnel: w359 -> [w361 w363]
                  tunnel: [w360 w362] -> w358
                  frame "Idle", Default {
                    n132 = call <vilib>:"Unset Busy.vi"("error in (no error)"=w361) -> ("error out"=w360:errorcluster)  [unwired: 10 in]
                  }
                  frame "Busy" {
                    n133 = call <vilib>:"Set Busy.vi"("error in (no error)"=w363) -> ("error out"=w362:errorcluster)  [unwired: 9 in, 1 out]
                  }
                }
              }
            }
            n134 = call <vilib>:"Add State(s) to Queue__jki_lib_state_machine.vi"("State(s) in (\"\")"=w355) -> ("States Out"=w354:string)  [unwired: 14 in]
          }
          frame "UI: Front Panel State" {
            # "Argument"
            # "Set Front Panel Open or Closed\n(Usage: \"UI: Front Panel State >> Open|Close\")"
            n135 = Unbundle By Name(w367) -> ("Core.Current VI Reference"=w366:refnum<vi>)
            n136 = disable-structure shown="Default" {
              disable-tunnel: w369 -> [w375 w398]
              disable-tunnel: [w374 w398] -> w368
              disable-tunnel: w366 -> [w373 _]
              disable-tunnel: w365 -> [w372 _]
              frame condition #0 (active) {
                n137 = case shown="\"Open\", Default" w372 {
                  tunnel: w375 -> [w379 w392]
                  tunnel: [w381 w393] -> w374
                  tunnel: w373 -> [w380 w390]
                  frame "Open", Default {
                    n138 = property class="VI"(reference=w380, error in=w379) -> (reference out=w377:refnum<vi>, error out=w378:errorcluster, "FP.State"=w376:T4)
                    n139 = case shown="\"Closed\"" w376 {
                      tunnel: [w384 w387] -> w381
                      tunnel: w378 -> [w383 w387]
                      tunnel: w377 -> [w382 _]
                      frame "Closed" {
                        n140 = invoke class="VI" method="FP.Open"(reference=w382, error in=w383, "Activate"=TRUE, "State"=T4."Standard") -> (error out=w384:errorcluster)  [unwired: 1 in, 4 out]
                      }
                      frame Default {
                      }
                    }
                  }
                  frame "Close" {
                    n141 = property class="VI"(reference=w390, error in=w392) -> (reference out=w389:refnum<vi>, error out=w391:errorcluster, "FP.State"=w388:T4)
                    n142 = case shown="Default" w388 {
                      tunnel: [w394 w397] -> w393
                      tunnel: w391 -> [w394 w396]
                      tunnel: w389 -> [_ w395]
                      frame "Invalid", "Closed" {
                      }
                      frame Default {
                        n143 = invoke class="VI" method="FP.Close"(reference=w395, error in=w396) -> (error out=w397:errorcluster)  [unwired: 1 in, 2 out]
                      }
                    }
                  }
                }
              }
              frame condition #1 {
              }
            }
            n144 = call <vilib>:"Add State(s) to Queue__jki_lib_state_machine.vi"("State(s) in (\"\")"=w371) -> ("States Out"=w370:string)  [unwired: 14 in]
          }
          frame "UI: Minimize" {
            # "Do not put any code in this frame.\n(It is a separator no-op. You can make a copy of this frame to create a new UI frame)"
            n145 = Unbundle By Name(w404) -> ("Core.Current VI Reference"=w403:refnum<vi>)
            n146 = property class="VI"(reference=w403, error in=w400) -> (reference out=w402:refnum<vi>, error out=w401:errorcluster, "Front Panel.PanelBounds"=w408:T9)
            n147 = case shown="\"Min\", Default" w406 {
              tunnel: w408 -> [w411 w419]
              tunnel: [w418 w426] -> w407
              frame "Min", Default {
                n148 = Unbundle By Name(w411) -> ("Left"=w417:i16, "Top"=w415:i16)
                n149 = Add(x=i16 776 ("x 6"), y=w417) -> (x+y=w416:i16)
                n150 = Add(x=w415, y=i16 184 ("x 5")) -> (x+y=w414:i16)
                n151 = Bundle By Name(cluster=w411, "Right"=w416, "Bottom"=w414) -> (w418:T9)
              }
              frame "Max" {
                n152 = Unbundle By Name(w419) -> ("Left"=w425:i16, "Top"=w423:i16)
                n153 = Add(x=i16 1168 ("x 8"), y=w425) -> (x+y=w424:i16)
                n154 = Add(x=w423, y=i16 584 ("x 7")) -> (x+y=w422:i16)
                n155 = Bundle By Name(cluster=w419, "Right"=w424, "Bottom"=w422) -> (w426:T9)
              }
            }
            n156 = property class="VI"(reference=w402, error in=w401, "Front Panel.PanelBounds"=w407) -> (error out=w399:errorcluster)  [unwired: 1 out]
            n157 = call <vilib>:"Add State(s) to Queue__jki_lib_state_machine.vi"("State(s) in (\"\")"=w405) -> ("States Out"=w410:string)  [unwired: 14 in]
          }
          frame "---------- Macro ----------" {
            # "Do not put any code in this frame.\n(It is a separator no-op. You can make a copy of this frame to create a new Macro frame)"
            n158 = call <vilib>:"Add State(s) to Queue__jki_lib_state_machine.vi"("State(s) in (\"\")"=w431) -> ("States Out"=w430:string)  [unwired: 14 in]
          }
          frame "Macro: Initialize" {
            w434 = "UI: Initialize\nUI: Front Panel State >> Open\nUI: Status 2 >> ..."  # UI: Initialize UI: Front Panel State >> Open UI: Status 2 >> ...
            # "Initialization Macro\n(This is called once, when the VI starts)"
            n159 = call <vilib>:"Add State(s) to Queue__jki_lib_state_machine.vi"("State(s) in Front (\"\")"="Data: Initialize\nInitialize Core Data\nEvents: Register", "State(s) in (\"\")"="Process: Sync", "State(s) at Back (\"\")"=w434) -> ("States Out"=w433:string)  [unwired: 12 in]
            n160 = call <vilib>:"Add State(s) to Queue__jki_lib_state_machine.vi"("State(s) in Front (\"\")"=w433, "State(s) in (\"\")"=w440) -> ("States Out"=w439:string)  [unwired: 13 in]
          }
          frame "Macro: Exit" {
            # "Exit Macro\n(This is called once, when the VI exits)"
            n161 = Unbundle By Name(w445) -> ("Core.Close Panel on Exit?"=w451:bool)
            n162 = Select(t="UI: Front Panel State >> Close", s=w451, f="") -> (s? t:f=w448:string)
            n163 = call <vilib>:"Add State(s) to Queue__jki_lib_state_machine.vi"("State(s) in Front (\"\")"="Data: Cleanup\nEvents: Unregister\nProcess: Self Terminate", "State(s) in (\"\")"="Process: Sync", "State(s) at Back (\"\")"="Exit") -> ("States Out"=w442:string)  [unwired: 12 in]
            n164 = call <vilib>:"Add State(s) to Queue__jki_lib_state_machine.vi"("State(s) in (\"\")"=w448, "State(s) at Back (\"\")"=w442) -> ("States Out"=w447:string)  [unwired: 13 in]
            n165 = call <vilib>:"Add State(s) to Queue__jki_lib_state_machine.vi"("State(s) in Front (\"\")"=w447, "State(s) in (\"\")"=w454) -> ("States Out"=w453:string)  [unwired: 13 in]
          }
          frame "---------- Process ----------" {
            # "Template Separator\n(You can make a copy of, or modify, this frame)"
            n166 = call <vilib>:"Add State(s) to Queue__jki_lib_state_machine.vi"("State(s) in (\"\")"=w459) -> ("States Out"=w458:string)  [unwired: 14 in]
          }
          frame "Process: Sync" {
            n167 = Unbundle By Name(w467) -> ("Instrument UI out"=w463:refnum<class "Instrument.OxfordVRM UI.lvclass">)
            n168 = call <vilib>:"WaitOnProcessSync.vi"("error in (no error)"=w462, "SMO"=w463) -> ("error out"=w461:errorcluster, "Don't run?"=w466:bool)  [unwired: 7 in, 1 out]
            n169 = Select(t="Data: Cleanup\nEvents: Unregister\nExit", s=w466, f="") -> (s? t:f=w460:string)
            n170 = call <vilib>:"Add State(s) to Queue__jki_lib_state_machine.vi"("State(s) in Front (\"\")"=w460, "State(s) in (\"\")"=w470) -> ("States Out"=w469:string)  [unwired: 13 in]
          }
          frame "Process: Self Terminate" {
            n171 = Unbundle By Name(w472) -> ("Instrument UI out"=w471:refnum<class "Instrument.OxfordVRM UI.lvclass">)
            n172 = call <vilib>:"SelfTerminate.vi"("error in (no error)"=w474, "SMO in"=w471) -> ("error out"=w473:errorcluster)  [unwired: 8 in, 1 out]
            n173 = call <vilib>:"Add State(s) to Queue__jki_lib_state_machine.vi"("State(s) in (\"\")"=w477) -> ("States Out"=w476:string)  [unwired: 14 in]
          }
          frame "---------- Events ----------" {
            # "Template Separator\n(You can make a copy of, or modify, this frame)"
            n174 = call <vilib>:"Add State(s) to Queue__jki_lib_state_machine.vi"("State(s) in (\"\")"=w482) -> ("States Out"=w481:string)  [unwired: 14 in]
          }
          frame "Events: Register" {
            # "Expand to add\nmore events"
            # "Base Class Protected Events"
            n175 = Unbundle By Name(w496) -> ("Instrument UI out"=w490:refnum<class "Instrument.OxfordVRM UI.lvclass">, "Instrument"=w488:refnum<class "Instrument.OxfordVRM.lvclass">)
            n176 = call <vilib>:"GetProtectedEvents.vi"("SMO"=w490) -> ("error out"=w491:errorcluster, "SMO Protected Events"=w494:T10)  [unwired: 8 in, 1 out]
            n177 = call <userlib>:"Instrument.GetPublicEvents.vi"("Instrument"=w488) -> ("error out"=w489:errorcluster, "Instrument Public Events"=w486:T11, "Instrument out"=w485:refnum<class "Instrument.OxfordVRM.lvclass">)  [unwired: 8 in]
            n178 = call "Instrument.Oxford1820.GetPublicEvents.vi"("Instrument.VRM in"=w485) -> ("error out"=w483:errorcluster, "VRM Public Events"=w484:T12)  [unwired: 8 in, 1 out]
            n179 = register-events(w494, w486, w484) -> (reference out=w495:refnum<event-registration>, error out=w493:errorcluster)  [unwired: 2 in]
            n180 = Merge Errors(w483, w489, w487, w493, w491) -> (w492:errorcluster)
            n181 = call <vilib>:"Add State(s) to Queue__jki_lib_state_machine.vi"("State(s) in (\"\")"=w498) -> ("States Out"=w497:string)  [unwired: 14 in]
          }
          frame "Events: Unregister" {
            n182 = Unregister For Events(event registration refnum=w501, error in=w500) -> (error out=w499:errorcluster)
            n183 = call <vilib>:"Add State(s) to Queue__jki_lib_state_machine.vi"("State(s) in (\"\")"=w504) -> ("States Out"=w503:string)  [unwired: 14 in]
          }
          frame "---------- Action ----------" {
            n184 = Unbundle By Name(w507) -> ("Instrument UI out"=w505:refnum<class "Instrument.OxfordVRM UI.lvclass">)
            n185 = Bundle By Name(cluster=w507, "Instrument UI out"=w505) -> (w506:T6)
            n186 = call <vilib>:"Add State(s) to Queue__jki_lib_state_machine.vi"("State(s) in (\"\")"=w511) -> ("States Out"=w510:string)  [unwired: 14 in]
          }
          frame "Action: Notify UI Closed" {
            # "Notify that the UI has been closed"
            n187 = Unbundle By Name(w514) -> ("Instrument UI out"=w515:refnum<class "Instrument.OxfordVRM UI.lvclass">)
            n188 = call <vilib>:"Hide.vi"("error in (no error)"=w513, "SMO.UI"=w515) -> ("error out"=w512:errorcluster)  [unwired: 8 in, 1 out]
            n189 = call <vilib>:"Add State(s) to Queue__jki_lib_state_machine.vi"("State(s) in (\"\")"=w518) -> ("States Out"=w517:string)  [unwired: 14 in]
          }
          frame "Action: get All" {
            n190 = Unbundle By Name(w519) -> ("Instrument"=w524:refnum<class "Instrument.OxfordVRM.lvclass">)
            n191 = call <userlib>:"Get ALL.vi"("error in (no error)"=w523, "Instrument in"=w524) -> ("error out"=w522:errorcluster, "getAll"=w520:variant, "Instrument out"=w521:refnum<class "Instrument.OxfordVRM.lvclass">)  [unwired: 7 in]
            n192 = Bundle By Name(cluster=w519, "Instrument"=w521, "getAll"=w520) -> (w525:T6)
            n193 = call <vilib>:"Add State(s) to Queue__jki_lib_state_machine.vi"("State(s) in (\"\")"=w528) -> ("States Out"=w527:string)  [unwired: 14 in]
          }
          frame "Action: Hold" {
            n194 = Unbundle By Name(w534) -> ("Instrument"=w532:refnum<class "Instrument.OxfordVRM.lvclass">)
            n195 = call "Instrument.Oxford1820.AbortSequence.vi"("error in (no error)"=w530, "Instrument.VRM in"=w532) -> ("error out"=w529:errorcluster, "Instrument.VRM out"=w531:refnum<class "Instrument.OxfordVRM.lvclass">)  [unwired: 8 in]
            n196 = call "Hold.vi"("error in (no error)"=w529, "Instrument.VRM in"=w531) -> ("error out"=w533:errorcluster)  [unwired: 7 in, 2 out]
            n197 = call <vilib>:"Add State(s) to Queue__jki_lib_state_machine.vi"("State(s) in (\"\")"=w537) -> ("States Out"=w536:string)  [unwired: 14 in]
          }
          frame "Action: To Zero" {
            n198 = Unbundle By Name(w541) -> ("Instrument"=w540:refnum<class "Instrument.OxfordVRM.lvclass">)
            n199 = call "Ramp to Zero.vi"("error in (no error)"=w539, "Instrument.VRM in"=w540) -> ("error out"=w538:errorcluster)  [unwired: 7 in, 2 out]
            n200 = call <vilib>:"Add State(s) to Queue__jki_lib_state_machine.vi"("State(s) in (\"\")"=w544) -> ("States Out"=w543:string)  [unwired: 14 in]
          }
          frame "Action: To Set" {
            n201 = Unbundle By Name(w548) -> ("Instrument"=w547:refnum<class "Instrument.OxfordVRM.lvclass">)
            n202 = call "Ramp to Set.vi"("error in (no error)"=w546, "Instrument.VRM in"=w547) -> ("error out"=w545:errorcluster)  [unwired: 7 in, 2 out]
            n203 = call <vilib>:"Add State(s) to Queue__jki_lib_state_machine.vi"("State(s) in (\"\")"=w551) -> ("States Out"=w550:string)  [unwired: 14 in]
          }
          frame "Action: Clamp" {
            n204 = Unbundle By Name(w552) -> ("Instrument"=w555:refnum<class "Instrument.OxfordVRM.lvclass">)
            n205 = call "Clamp.vi"("error in (no error)"=w554, "Instrument.VRM in"=w555) -> ("error out"=w553:errorcluster)  [unwired: 7 in, 2 out]
            n206 = call <vilib>:"Add State(s) to Queue__jki_lib_state_machine.vi"("State(s) in (\"\")"=w558) -> ("States Out"=w557:string)  [unwired: 14 in]
          }
          frame "Action: Send to IPS" {
            n207 = Unbundle By Name(w564) -> ("Instrument"=w563:refnum<class "Instrument.OxfordVRM.lvclass">)
            n208 = call "Set Target.vi"("error in (no error)"=w560, "Target Rate (T/min)"="Target Rate (T/min)", "Target Field (T)"="Target Field (T)", "Instrument.VRM in"=w563) -> ("error out"=w559:errorcluster)  [unwired: 5 in, 2 out]
            n209 = call <vilib>:"Add State(s) to Queue__jki_lib_state_machine.vi"("State(s) in (\"\")"=w567) -> ("States Out"=w566:string)  [unwired: 14 in]
          }
        }
      }
    }
    frame Error {
    }
  }
  n210 = call-parent "Process.vi"("error in"=w12, "Instrument UI in"=w11) -> ("error out"=w9:errorcluster, "Instrument UI out"=→"Instrument.OxfordVRM UI.lvclass":refnum<class "Instrument.OxfordVRM UI.lvclass">)  [unwired: 8 in]
  n211 = disable-structure shown="Disabled" {
    frame Disabled {
    }
    frame Enabled {
    }
  }
  n212 = Merge Errors(w9, w8) -> (→"error out":errorcluster)
  n213 = local read "Target Rate (T/min)"() -> (w3:dbl)
  n214 = call "VRM Cartesian to Spherical.vi"("Field (x,y,z)"="Setpoint (T)") -> ("Field (r,theta,phi)"=→"Setpoint (T) (sph)":dbl[])  [unwired: 9 in, 1 out]
  n215 = call "VRM Calculate Sweep Rates.vi"("Sweep rate (T/min)"=w3) -> ()  [unwired: 8 in, 3 out]
  "version" <- "v20/12/08" ("version")
